vi "Rename Object.vi"(4 "Post":string, 6 "Pre":string, 8 "error in":errorcluster, 9 "Rename Library File Path":path, 10 "Project:Active Project":refnum<vi>) -> (0 "error out":errorcluster, 2 "Object Ref":refnum<vi>)   [LabVIEW 2020, in "_Rename.lvlib" / "_Rename.lvclass"]
uses:
  _Rename.lvclass
  <vilib>/Utility/EditLVLibs/Edit LVLibs.lvlib
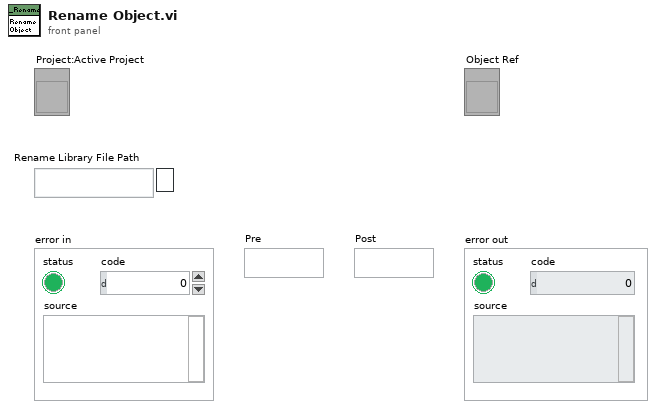
[diagram p1: front panel]
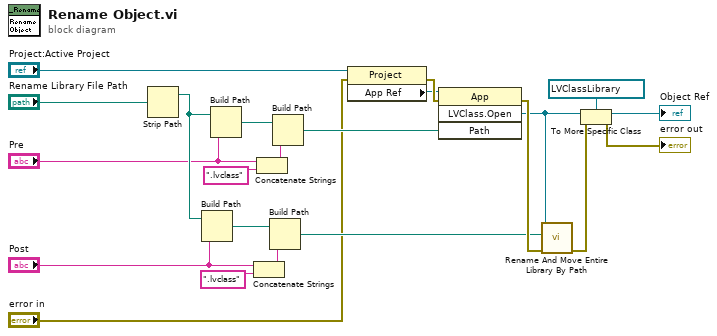
[diagram p0: block diagram]
diagram:
  n1 = Strip Path(path="Rename Library File Path") -> (stripped path=w8:path)  [unwired: 1 out]
  n2 = Build Path(base path=w8, name or relative path="Post") -> (appended path=w14:path)
  n3 = Build Path(base path=w8, name or relative path="Pre") -> (appended path=w10:path)
  n4 = Concatenate Strings("Post", ".lvclass" ("string")) -> (w16:string)
  n5 = Concatenate Strings("Pre", ".lvclass" ("string")) -> (w12:string)
  n6 = Build Path(base path=w14, name or relative path=w16) -> (appended path=w13:path)
  n7 = Build Path(base path=w10, name or relative path=w12) -> (appended path=w9:path)
  n8 = property class="Project"(reference="Project:Active Project", error in="error in") -> (error out=w21:errorcluster, "App Ref"=w20:refnum<vi>)  [unwired: 1 out]
  n9 = invoke class="App" method="LVClass.Open"(reference=w20, error in=w21, "Path"=w9) -> (error out=w22:errorcluster, "LVClass.Open"=w18:refnum<vi>)  [unwired: 1 in, 2 out]
  n10 = call <vilib>:"Rename And Move Entire Library By Path.vi"("error in (no error)"=w22, "New library path"=w13, "Library ref in"=w18) -> ("error out"=w17:errorcluster)  [unwired: 7 in, 1 out]
  n11 = To More Specific Class(target class=refnum<vi> refnum ("Class in"), reference=w18, error in=w17) -> (specific class reference=→"Object Ref":refnum<vi>, error out=→"error out":errorcluster)
